vi "RFFE Write_Read_Cmd.vi"(8 "error in":errorcluster, 10 "Cmd":string, 11 "VISA In":refnum<visa-resource-name>) -> (0 "error out":errorcluster, 2 "read buffer":string, 3 "VISA Out":refnum<visa-resource-name>)   [LabVIEW 2017]
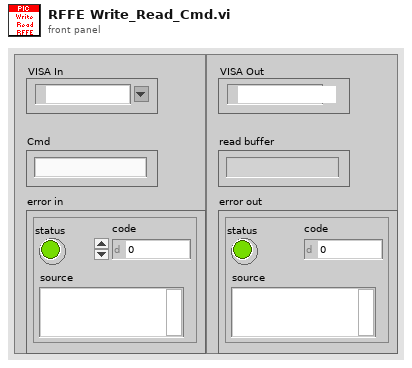
[diagram p1: front panel]
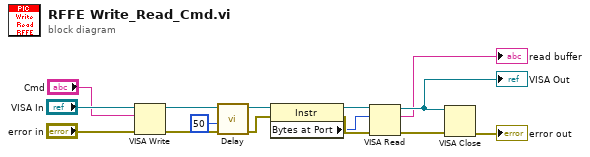
[diagram p0: block diagram]
diagram:
  n1 = VISA Write(VISA resource name="VISA In", write buffer="Cmd", error in (no error)="error in") -> (VISA resource name out=w8:refnum<visa-resource-name>, error out=w14:errorcluster)  [unwired: 1 out]
  n2 = call "Delay.vi"("error in (no error)"=w14, "Delay"=u32 50) -> ("error out"=w9:errorcluster)  [unwired: 9 in]
  n3 = property class="Instr"(reference=w8, error in=w9) -> (reference out=w7:refnum<visa-resource-name>, error out=w10:errorcluster, "Bytes at Port"=w6:u32)
  n4 = VISA Read(VISA resource name=w7, byte count=w6, error in (no error)=w10) -> (VISA resource name out=w5:refnum<visa-resource-name>, read buffer=→"read buffer":string, error out=w4:errorcluster)  [unwired: 1 out]
  "VISA Out" <- w5
  n5 = VISA Close(VISA resource name=w5, error in (no error)=w4) -> (error out=→"error out":errorcluster)
